vi "TOD Byte Stream to String.vi"(8 "error in (no error)":errorcluster, 10 "Byte Stream":u8[](array[numeric])) -> (0 "error out":errorcluster, 2 "Value":string)   [LabVIEW 2018, in "TwinCAT ADS.lvclass"]
uses:
  TwinCAT ADS.lvclass
  TwinCAT.Ads
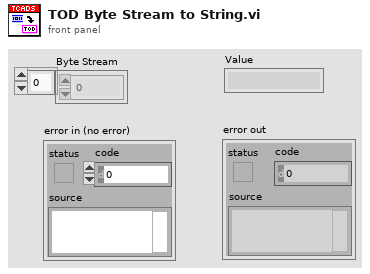
[diagram p1: front panel]
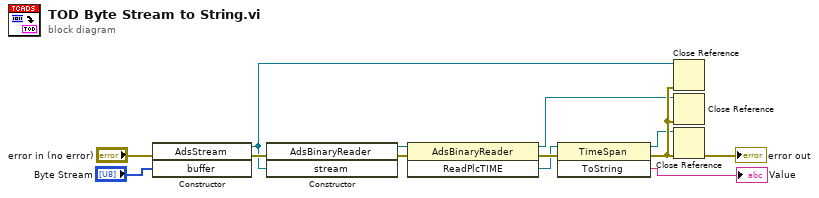
[diagram p0: block diagram]
diagram:
  n1 = constructor class="AdsStream"(error in="error in (no error)", "buffer"="Byte Stream") -> (reference out=w5:refnum<k24>, error out=w13:errorcluster)  [unwired: 2 in, 2 out]
  n2 = constructor class="AdsBinaryReader"(error in=w13, "stream"=w5) -> (reference out=w11:refnum<k24>, error out=w12:errorcluster)  [unwired: 2 in, 2 out]
  n3 = invoke class="AdsBinaryReader" method="ReadPlcTIME"(reference=w11, error in=w12) -> (reference out=w6:refnum<k24>, error out=w10:errorcluster, "ReadPlcTIME"=w9:refnum<k24>)  [unwired: 1 in]
  n4 = invoke class="TimeSpan" method="ToString"(reference=w9, error in=w10) -> (reference out=w7:refnum<k24>, error out=w8:errorcluster, "ToString"=→"Value":string)  [unwired: 1 in]
  n5 = Close Reference(reference=w5, error in (no error)=w8) -> ()  [unwired: 1 out]
  n6 = Close Reference(reference=w6, error in (no error)=w8) -> ()  [unwired: 1 out]
  n7 = Close Reference(reference=w7, error in (no error)=w8) -> (error out=→"error out":errorcluster)
